vi "Write Spreadsheet Message.vi"(8 "error in (no error)":errorcluster, 10 "Acquired Data":T12, 11 "Settings":T1) -> (0 "error out":errorcluster, 3 "Settings":T1)   [LabVIEW 2021, in "Logging.lvlib"]
doc: "Write 'Acquired Data' to the data log file, using the first channel's timestamp for the first column and each channel's measurement for the remaining columns."
uses:
  Logging.lvlib
  Acquisition/Acquired Data.ctl
  Settings/Settings.ctl
  Acquisition/Hardware Configuration.ctl
  Acquisition/Channel Settings.ctl
  Acquisition/IO Device.ctl
  Interval Timer/Repeat Interval.ctl
  Interval Timer/Interval Length.ctl
  Interval Timer/Interval Token.ctl
  Acquisition/IO API.ctl
  Logging Configuration.ctl
  Logging Mode.ctl
  Diagnostics/Diagnostics Configuration.ctl
  Acquisition/Acquisition.lvlib
  Settings/Settings.lvlib
  Diagnostics/Diagnostics.lvlib
  Interval Timer/Interval Timer.lvlib
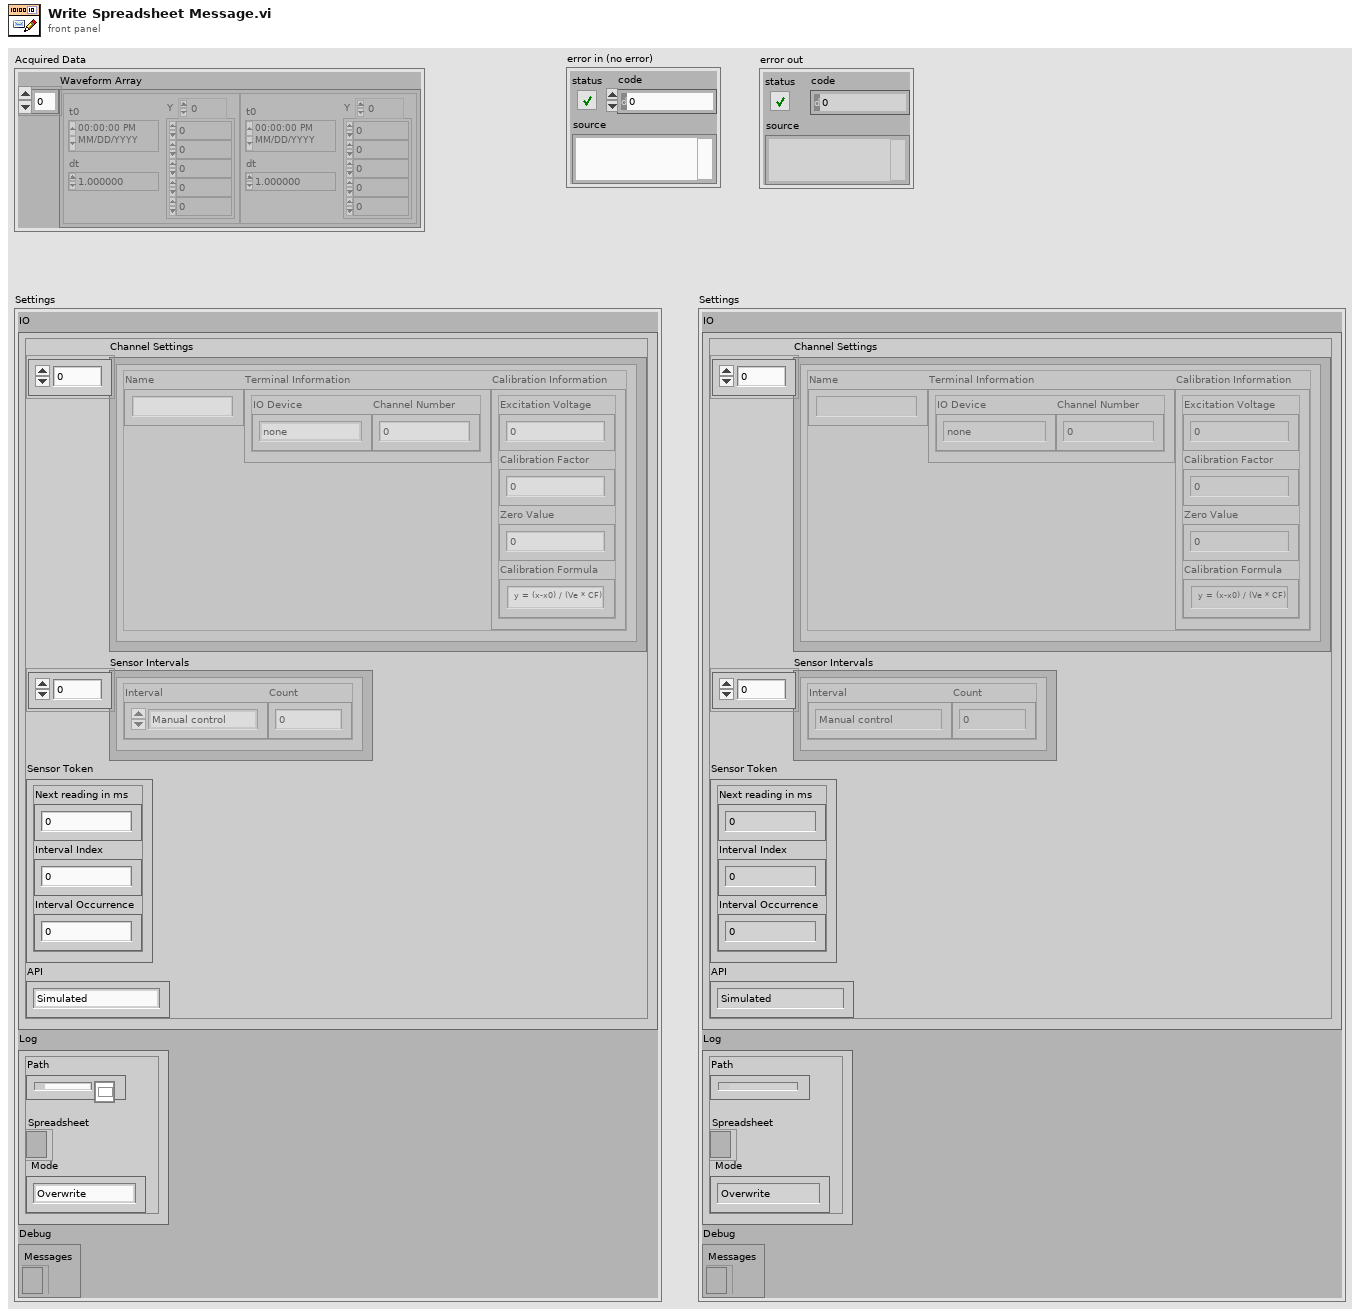
[diagram p1: front panel]
types:
  T1 = typedef "Settings.lvlib/Settings.ctl" = cluster{"IO":T2, "Log":T9, "Debug":T11}
  T2 = typedef "Acquisition.lvlib/Hardware Configuration.ctl" = cluster{"Channel Settings":T3[], "Sensor Intervals":T5[], "Sensor Token":T7, "API":T8}
  T3 = typedef "Acquisition.lvlib/Channel Settings.ctl" = cluster{"Name":string, "Terminal Information":cluster{"IO Device":T4, "Channel Number":i32}, "Calibration Information":cluster{"Excitation Voltage":dbl, "Calibration Factor":dbl, "Zero Value":dbl, "Calibration Formula":string}}
  T4 = typedef "Acquisition.lvlib/IO Device.ctl" = enum16{"none", "9219", "9401"}
  T5 = typedef "Interval Timer.lvlib/Repeat Interval.ctl" = cluster{"Interval":T6, "Count":i32}
  T6 = typedef "Interval Timer.lvlib/Interval Length.ctl" = enum16{"Manual control", "1 second", "10 seconds", "30 seconds", "60 seconds", "600 seconds", "1200 seconds", "3600 seconds"}
  T7 = typedef "Interval Timer.lvlib/Interval Token.ctl" = cluster{"Next reading in ms":u32, "Interval Index":i32, "Interval Occurrence":i32}
  T8 = typedef "Acquisition.lvlib/IO API.ctl" = enum16{"Simulated", "DAQmx"}
  T9 = typedef "Logging.lvlib/Logging Configuration.ctl" = cluster{"Path":path, "Spreadsheet":refnum<file>, "Mode":T10}
  T10 = typedef "Logging.lvlib/Logging Mode.ctl" = enum16{"Overwrite", "Append", "Create New"}
  T11 = typedef "Diagnostics.lvlib/Diagnostics Configuration.ctl" = cluster{"Messages":refnum<file>}
  T12 = typedef "Acquisition.lvlib/Acquired Data.ctl" = cluster{"Waveform Array":waveform(dbl)[]}
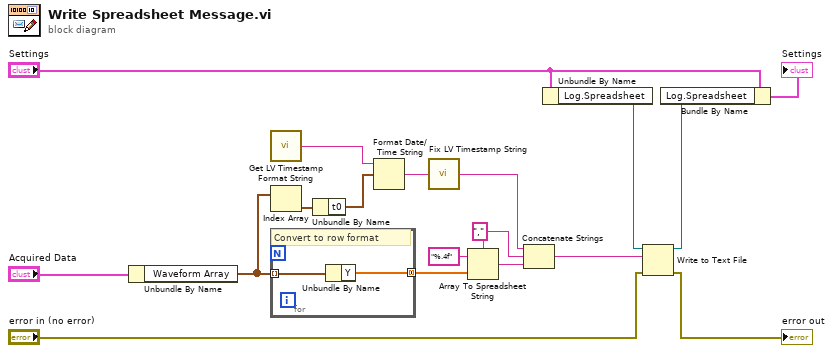
[diagram p0: block diagram]
diagram:
  w7 = "," ("delimiter (Tab)")
  n1 = Unbundle By Name("Acquired Data") -> ("Waveform Array"=w6:waveform(dbl)[])
  n2 = call "Get LV Timestamp Format String.vi"() -> ("timestamp string format"=w3:string)
  n3 = Index Array(array=w6) -> (element=w5:waveform(dbl))  [unwired: 1 in]
  n4 = for {
    tunnel: w6 -> [w20] mode=indexing
    tunnel: [w19] -> w11 mode=concatenating
    # "Convert to row format"
    n5 = Unbundle By Name(w20) -> ("Y"=w19:dbl[])
  }
  n6 = Unbundle By Name(w5) -> ("t0"=w4:timestamp)
  n7 = Format Date/Time String(time format string (%c)=w3, seconds (now)=w4) -> (date/time string=w2:string)  [unwired: 1 in]
  n8 = call "Fix LV Timestamp String.vi"("LabVIEW format string"=w2) -> ("iso 8601 format string"=w1:string)
  n9 = Array To Spreadsheet String(delimiter (Tab)=w7, array=w11, 3:"%.4f" ("format string")) -> (spreadsheet string=w9:string)
  n10 = Concatenate Strings(w1, w7, w9) -> (w8:string)
  n11 = Unbundle By Name("Settings") -> ("Log.Spreadsheet"=w14:refnum<file>)
  n12 = Write to Text File(file (use dialog)=w14, text=w8, error in="error in (no error)") -> (refnum out=w12:refnum<file>, error out=→"error out":errorcluster)  [unwired: 1 in, 1 out]
  n13 = Bundle By Name(cluster="Settings", "Log.Spreadsheet"=w12) -> (→"Settings":T1)
